vi "loadcolormaps.vi"   [LabVIEW 2015]
uses:
  <vilib>/Utility/file.llb/Read Delimited Spreadsheet (DBL).vi
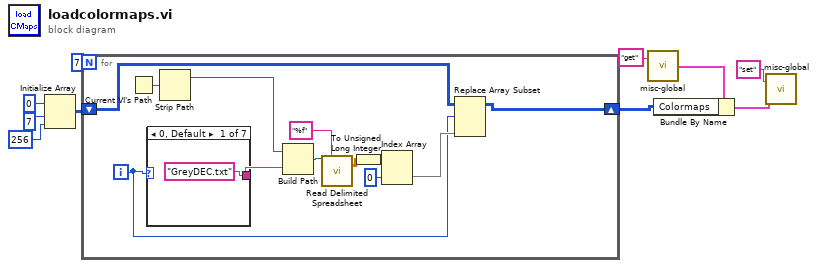
[diagram p0: block diagram]
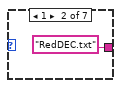
[diagram p2: hidden frame]
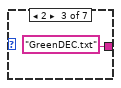
[diagram p3: hidden frame]
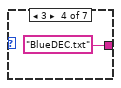
[diagram p4: hidden frame]
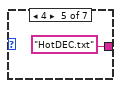
[diagram p5: hidden frame]
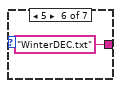
[diagram p6: hidden frame]
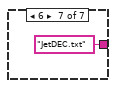
[diagram p7: hidden frame]
diagram:
  n1 = Initialize Array(u32 0 ("element"), 7 ("dimension size"), 256 ("dimension size")) -> (w5:u32[][])
  n2 = for {
    N: 7 -> [_]
    shift-right: [w14] -> w8
    shift-left: w5 -> [w16]
    i -> [w13]
    n3 = Current VI's Path() -> (path=w22:path)
    n4 = case shown="0, Default" w13 {
      tunnel: ["GreyDEC.txt" "RedDEC.txt" "GreenDEC.txt" "BlueDEC.txt" "HotDEC.txt" "WinterDEC.txt" "JetDEC.txt"] -> w21
      frame 0, Default {
      }
      frame 1 {
      }
      frame 2 {
      }
      frame 3 {
      }
      frame 4 {
      }
      frame 5 {
      }
      frame 6 {
      }
    }
    n5 = Strip Path(path=w22) -> (stripped path=w11:path)  [unwired: 1 out]
    n6 = Build Path(base path=w11, name or relative path=w21) -> (appended path=w17:path)
    n7 = call-poly <vilib>:"Read Delimited Spreadsheet.vi"("file path (dialog if empty)"=w17, "format (%.3f)"="%f") -> ("all rows"=w19:dbl[][])  [unwired: 8 in, 5 out]
    n8 = To Unsigned Long Integer(number=w19) -> (unsigned 32bit integer=w12:u32[][])
    n9 = Index Array(array=w12, index (col)=0 ("disabled index (col)")) -> (element=w15:u32[])  [unwired: 1 in]
    n10 = Replace Array Subset(array=w16, new element=w15, index (row)=w13) -> (w14:u32[][])  [unwired: 1 in]
  }
  n11 = call "misc-global.vi"("command"="get") -> ("misc out"=w7:cluster{"Colormaps":u32[][]})  [unwired: 1 in]
  n12 = Bundle By Name(cluster=w7, "Colormaps"=w8) -> (w10:cluster{"Colormaps":u32[][]})
  n13 = call "misc-global.vi"("misc in"=w10, "command"="set") -> ()  [unwired: 1 out]
